vi "KeyboardToJoystick.vi"(8 "LeftRightValue":dbl=0.75, 9 "UpDownValue":dbl=0.75) -> (1 "Turn":dbl, 2 "Throttle":dbl)   [LabVIEW 2018]
uses:
  <vilib>/Utility/inputDevices.llb/closeJoystick.vi
  Robot Global Data.vi
  <vilib>/Utility/inputDevices.llb/keyboardAcquire.vi
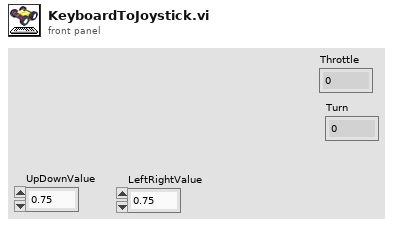
[diagram p1: front panel]
types:
  T1 = enum16{"0", "1", "2", "3", "4", "5", "6", "7", "8", "9", "A", "B", "C", "D", "E", "F", "G", "H", "I", "J", "K", "L", "M", "N", "O", "P", "Q", "R", "S", "T", "U", "V", "W", "X", "Y", "Z", "F1", "F2", "F3", "F4", "F5", "F6", "F7", "F8", "F9", "F10", "F11", "F12", "F13", "F14", "F15", "ADD", "BACK", "BACKSLASH", "CAPITAL", "COMMA", "DECIMAL", "DELETE", "DIVIDE", "DOWN", "END", "EQUALS", "ESCAPE", "GRAVE (`)", "HOME", "INSERT", "LBRACKET", "LCONTROL", "LEFT", "L ALT", "LSHIFT", "LWIN", "MINUS", "MULTIPLY", "NEXT", "NUMLOCK", "NUMPAD_0", "NUMPAD_1", "NUMPAD_2", "NUMPAD_3", "NUMPAD_4", "NUMPAD_5", "NUMPAD_6", "NUMPAD_7", "NUMPAD_8", "NUMPAD_9", "PAUSE", "PERIOD", "PRIOR (PG UP)", "RBRACKET", "RCONTROL", "RETURN", "RIGHT", "R ALT", "RSHIFT", "RWIN", "SCROLL", "SEMICOLON", "SLASH", "SPACE", "SUBTRACT", "TAB", "UP", "ENTER (num pad)", "' (quote)"}[]
  T2 = enum16{"0", "1", "2", "3", "4", "5", "6", "7", "8", "9", "A", "B", "C", "D", "E", "F", "G", "H", "I", "J", "K", "L", "M", "N", "O", "P", "Q", "R", "S", "T", "U", "V", "W", "X", "Y", "Z", "F1", "F2", "F3", "F4", "F5", "F6", "F7", "F8", "F9", "F10", "F11", "F12", "F13", "F14", "F15", "ADD", "BACK", "BACKSLASH", "CAPITAL", "COMMA", "DECIMAL", "DELETE", "DIVIDE", "DOWN", "END", "EQUALS", "ESCAPE", "GRAVE (`)", "HOME", "INSERT", "LBRACKET", "LCONTROL", "LEFT", "L ALT", "LSHIFT", "LWIN", "MINUS", "MULTIPLY", "NEXT", "NUMLOCK", "NUMPAD_0", "NUMPAD_1", "NUMPAD_2", "NUMPAD_3", "NUMPAD_4", "NUMPAD_5", "NUMPAD_6", "NUMPAD_7", "NUMPAD_8", "NUMPAD_9", "PAUSE", "PERIOD", "PRIOR (PG UP)", "RBRACKET", "RCONTROL", "RETURN", "RIGHT", "R ALT", "RSHIFT", "RWIN", "SCROLL", "SEMICOLON", "SLASH", "SPACE", "SUBTRACT", "TAB", "UP", "ENTER (num pad)", "' (quote)"}
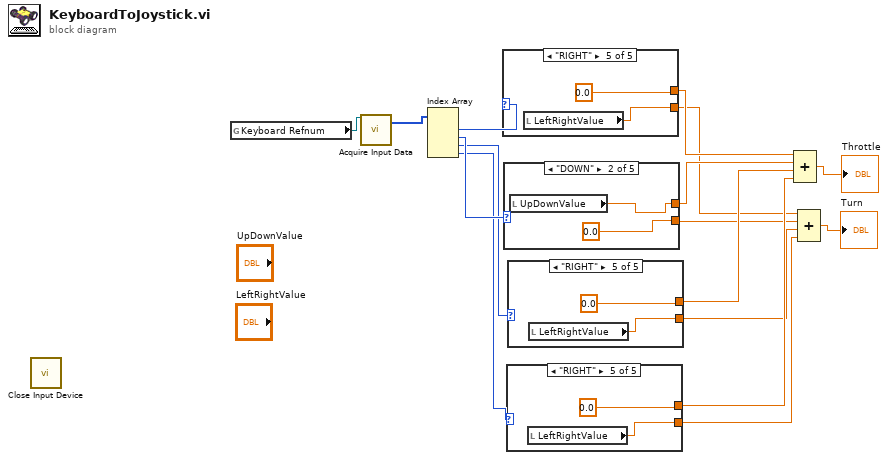
[diagram p0: block diagram]
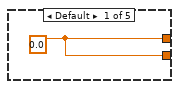
[diagram p2: hidden frame]
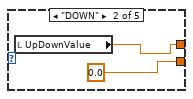
[diagram p3: hidden frame]
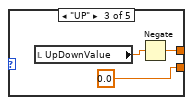
[diagram p4: hidden frame]
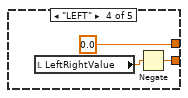
[diagram p5: hidden frame]
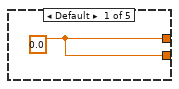
[diagram p6: hidden frame]
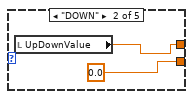
[diagram p7: hidden frame]
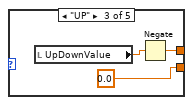
[diagram p8: hidden frame]
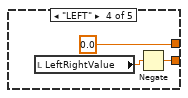
[diagram p9: hidden frame]
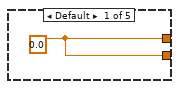
[diagram p10: hidden frame]
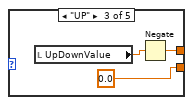
[diagram p11: hidden frame]
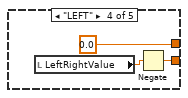
[diagram p12: hidden frame]
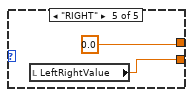
[diagram p13: hidden frame]
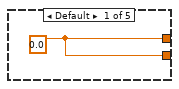
[diagram p14: hidden frame]
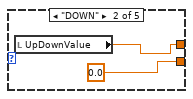
[diagram p15: hidden frame]
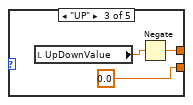
[diagram p16: hidden frame]
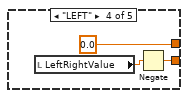
[diagram p17: hidden frame]
diagram:
  n1 = call-poly <vilib>:"Close Input Device.vi"() -> ()  [unwired: 10 in, 1 out]
  n2 = global read "Robot Global Data.vi" "Keyboard Refnum"() -> (w1:refnum<k1>)
  n3 = call-poly <vilib>:"Acquire Input Data.vi"("device ID"=w1) -> ("keys pressed"=w16:T1)  [unwired: 16 in, 2 out]
  n4 = Index Array(array=w16) -> (element #1=w15:T2, element #2=w11:T2, element #3=w10:T2, element #4=w9:T2)  [unwired: 4 in]
  n5 = case shown="\"RIGHT\"" w15 {
    tunnel: [w17 w18 w22 0.0 0.0] -> w12
    tunnel: [w17 0.0 0.0 w25 w27] -> w2
    frame Default {
      w17 = 0.0
    }
    frame "DOWN" {
      n6 = local read "UpDownValue"() -> (w18:dbl)
    }
    frame "UP" {
      n7 = local read "UpDownValue"() -> (w21:dbl)
      n8 = Negate(x=w21) -> (-x=w22:dbl)
    }
    frame "LEFT" {
      n9 = local read "LeftRightValue"() -> (w24:dbl)
      n10 = Negate(x=w24) -> (-x=w25:dbl)
    }
    frame "RIGHT" {
      n11 = local read "LeftRightValue"() -> (w27:dbl)
    }
  }
  n12 = case shown="\"DOWN\"" w11 {
    tunnel: [w28 w29 w33 0.0 0.0] -> w8
    tunnel: [w28 0.0 0.0 w36 w38] -> w3
    frame Default {
      w28 = 0.0
    }
    frame "DOWN" {
      n13 = local read "UpDownValue"() -> (w29:dbl)
    }
    frame "UP" {
      n14 = local read "UpDownValue"() -> (w32:dbl)
      n15 = Negate(x=w32) -> (-x=w33:dbl)
    }
    frame "LEFT" {
      n16 = local read "LeftRightValue"() -> (w35:dbl)
      n17 = Negate(x=w35) -> (-x=w36:dbl)
    }
    frame "RIGHT" {
      n18 = local read "LeftRightValue"() -> (w38:dbl)
    }
  }
  n19 = case shown="\"RIGHT\"" w9 {
    tunnel: [w39 w40 w44 0.0 0.0] -> w6
    tunnel: [w39 0.0 0.0 w47 w49] -> w5
    frame Default {
      w39 = 0.0
    }
    frame "DOWN" {
      n20 = local read "UpDownValue"() -> (w40:dbl)
    }
    frame "UP" {
      n21 = local read "UpDownValue"() -> (w43:dbl)
      n22 = Negate(x=w43) -> (-x=w44:dbl)
    }
    frame "LEFT" {
      n23 = local read "LeftRightValue"() -> (w46:dbl)
      n24 = Negate(x=w46) -> (-x=w47:dbl)
    }
    frame "RIGHT" {
      n25 = local read "LeftRightValue"() -> (w49:dbl)
    }
  }
  n26 = case shown="\"RIGHT\"" w10 {
    tunnel: [w50 w51 w55 0.0 0.0] -> w7
    tunnel: [w50 0.0 0.0 w58 w60] -> w4
    frame Default {
      w50 = 0.0
    }
    frame "DOWN" {
      n27 = local read "UpDownValue"() -> (w51:dbl)
    }
    frame "UP" {
      n28 = local read "UpDownValue"() -> (w54:dbl)
      n29 = Negate(x=w54) -> (-x=w55:dbl)
    }
    frame "LEFT" {
      n30 = local read "LeftRightValue"() -> (w57:dbl)
      n31 = Negate(x=w57) -> (-x=w58:dbl)
    }
    frame "RIGHT" {
      n32 = local read "LeftRightValue"() -> (w60:dbl)
    }
  }
  n33 = Compound Arithmetic op=ADD(w12, w8, w7, w6) -> (→"Throttle":dbl)
  n34 = Compound Arithmetic op=ADD(w2, w3, w4, w5) -> (→"Turn":dbl)
